vi "LoadArmValues.vi"(8 "error in (no error)":errorcluster, 11 "Robot":T1) -> (0 "error out":errorcluster)   [LabVIEW 2015]
uses:
  LowShooter/Implementation/Shooter Settings Type Def.ctl
  Drive/Implementation/Advanced Drive VIs/PID Type Def.ctl
  Arm/Arm Settings Type Def.ctl
  Robot Type Def.ctl
  <vilib>/Rock Robotics/Network Tables/NT Read Numeric Array.vi
  LowShooter/Implementation/Shooter Global.vi
panel:
  out "Arm Settings":T2
  out "PID":T3
  out "Shooter Settings":T4
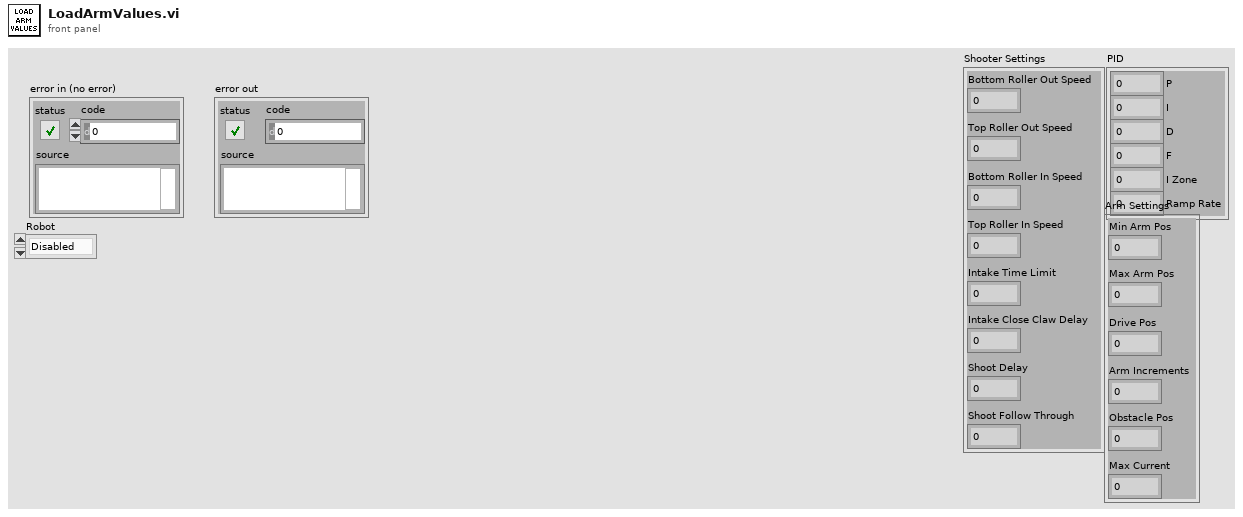
[diagram p1: front panel]
types:
  T1 = typedef "Robot Type Def.ctl" = enum32{"Disabled", "Ghost", "Casper", "Lofty", "Board", "RaceRobot", "Casper 2.0", "Excalibot 2.0"}
  T2 = typedef "Arm Settings Type Def.ctl" = cluster{"Min Arm Pos":dbl, "Max Arm Pos":dbl, "Drive Pos":dbl, "Arm Increments":dbl, "Obstacle Pos":dbl, "Max Current":dbl}
  T3 = typedef "PID Type Def.ctl" = cluster{"P":dbl, "I":dbl, "D":dbl, "F":dbl, "I Zone":dbl, "Ramp Rate":dbl}
  T4 = typedef "Shooter Settings Type Def.ctl" = cluster{"Bottom Roller Out Speed":dbl, "Top Roller Out Speed":dbl, "Bottom Roller In Speed":dbl, "Top Roller In Speed":dbl, "Intake Time Limit":dbl, "Intake Close Claw Delay":dbl, "Shoot Delay":dbl, "Shoot Follow Through":dbl}
  T5 = typedef "Detailed Motor Type Def.ctl" = cluster{"MotorRef":T6, "Encoder Ticks Per Rev":dbl, "Set Position":dbl, "Wheel Radius":dbl}
  T6 = typedef "WPI_MotorControlDeviceRef.ctl" = cluster{"DeviceStatus":errorcluster, "Type":T7, "PWM":cluster{"PWM Channel":T8, "DeadBand":T9}, "CAN":cluster{"Device Number":u8, "Control Mode":T10, "Semaphore":T11, "Max Vout":dbl, "TalonSRX Control Mode":T12}, "Invert":bool}
  T7 = typedef "WPI_MotorControlType.ctl" = enum16{"PWM", "CAN", "CANTalonSRX"}
  T8 = typedef "FPGA_DIOPWMChannel.ctl" = enum8{"PWM 0", "PWM 1", "PWM 2", "PWM 3", "PWM 4", "PWM 5", "PWM 6", "PWM 7", "PWM 8", "PWM 9", "PWM MXP 0", "PWM MXP 1", "PWM MXP 2", "PWM MXP 3", "PWM MXP 4", "PWM MXP 5", "PWM MXP 6", "PWM MXP 7", "PWM MXP 8", "PWM MXP 9", "Invalid"}
  T9 = typedef "WPI_PWMDeadband.ctl" = cluster{"Name":string, "maxPositivePwm":i32, "minPositivePwm":i32, "centerPwm":i32, "maxNegativePwm":i32, "minNegativePwm":i32, "angularRange":u16}
  T10 = typedef "WPI_CANJaguar_ControlMode.ctl" = enum8{"Percent VBus", "Current", "Speed", "Position", "Voltage"}
  T11 = typedef "Semaphore RefNum" = refnum<k1>
  T12 = typedef "WPI_CANTalonSRX_APIControlMode.ctl" = enum8{"Percent VBus", "Speed", "Position", "Slave", "Unchanged / Invalid", "Voltage Compensation", "Current", "Motion Profile"}
  T13 = typedef "WPI_CANTalonSRX_GlobalStatus.ctl" = cluster{"Applied Throttle":dbl, "Module Enabled":bool, "CAN Error":errorcluster, "Closed Loop Error":dbl, "Forward Limit Switch Closed":bool, "Reverse Limit Switch Closed":bool, "Sensor Position":dbl, "Sensor Velocity":dbl, "Current":dbl, "Sticky Fault - Over Temp":bool, "Sticky Fault - Under Voltage":bool, "Sticky Fault - Forward Limit":bool, "Sticky Fault - Reverse Limit":bool, "Sticky Fault - Forward Soft Limit":bool, "Sticky Fault - Reverse Soft Limit":bool, "Brake is Enabled":bool, "Encoder Position":dbl, "Encoder Velocity":dbl, "Encoder Index Count":dbl, "Encoder A Pin State":bool, "Encoder B Pin State":bool, "Encoder Index Pin State":bool, "Analog In":dbl, "Analog In Velocity":dbl, "Temperature (C)":dbl, "Battery Voltage":dbl, "Control 5 Is Supported":bool, "Current Profile Slot Select":dbl, "Pos Div 8":bool, "Vel Div 4":bool, "Pulse Width Position":i32, "Pulse Width Velocity":i32, "Pulse Width Rise To Rise (us)":i32, "Pulse Width Rise To Fall (us)":i32, "Mot Prof Active Is Under Run":bool, "Mot Prof Active Has Under Run":bool, "Mot Prof Active Is Last":bool, "Mot Prof Active Velocity Only":bool, "Mot Prof Active Is Valid":bool, "Mot Prof Buffer Is Full":bool, "Mot Prof Active Profile Slot Select":i32, "Mot Prof NextID":i32, "Mot Prof Count":i32, "Mot Prof Active Velocity":dbl, "Mot Prof Active Position":dbl, "Mot Prof Output Enable":i32}
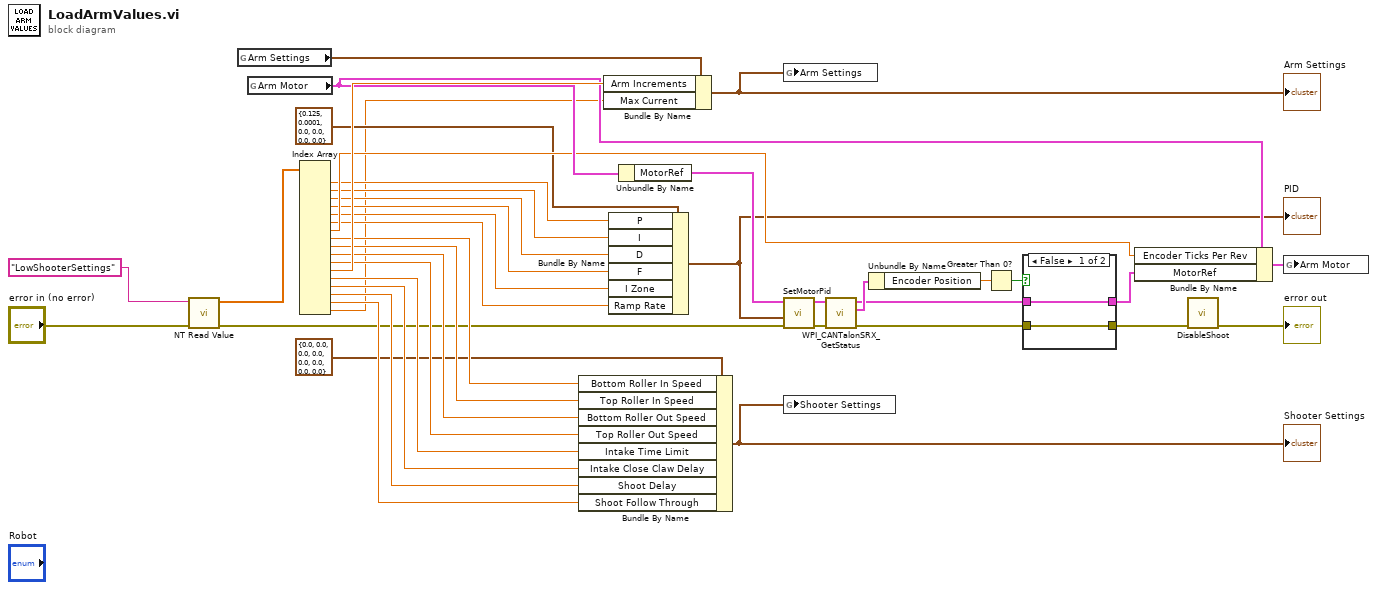
[diagram p0: block diagram]
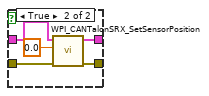
[diagram p2: hidden frame]
diagram:
  n1 = call-poly <vilib>:"NT Read Value.vi"("error in"="error in (no error)", "Name"="LowShooterSettings") -> ("error out"=w12:errorcluster, "Numeric Array"=w23:dbl[])  [unwired: 8 in]
  n2 = global read "Shooter Global.vi" "Arm Settings"() -> (w40:T2)
  n3 = global read "Shooter Global.vi" "Arm Motor"() -> (w36:T5)
  n4 = Index Array(array=w23) -> (element #1=w16:dbl, element #2=w17:dbl, element #3=w18:dbl, element #4=w19:dbl, element #5=w20:dbl, element #6=w21:dbl, element #7=w27:dbl, element #8=w28:dbl, element #9=w29:dbl, element #10=w30:dbl, element #11=w31:dbl, element #12=w38:dbl, element #13=w32:dbl, element #14=w33:dbl, element #15=w34:dbl, element #16=w35:dbl, element #17=w11:dbl)  [unwired: 17 in]
  n5 = Bundle By Name(cluster=T4 {"Bottom Roller Out Speed"=0.0, "Top Roller Out Speed"=0.0, "Bottom Roller In Speed"=0.0, "Top Roller In Speed"=0.0, "Intake Time Limit"=0.0, "Intake Close Claw Delay"=0.0, "Shoot Delay"=0.0, "Shoot Follow Through"=0.0} ("Shooter Settings"), "Bottom Roller In Speed"=w28, "Top Roller In Speed"=w29, "Bottom Roller Out Speed"=w30, "Top Roller Out Speed"=w31, "Intake Time Limit"=w32, "Intake Close Claw Delay"=w33, "Shoot Delay"=w34, "Shoot Follow Through"=w35) -> (w26:T4)
  "Shooter Settings" <- w26
  n6 = Bundle By Name(cluster=w40, "Arm Increments"=w38, "Max Current"=w11) -> (w39:T2)
  "Arm Settings" <- w39
  n7 = Bundle By Name(cluster=T3 {"P"=0.125, "I"=0.0001, "D"=0.0, "F"=0.0, "I Zone"=0.0, "Ramp Rate"=0.0} ("PID"), "P"=w16, "I"=w17, "D"=w18, "F"=w19, "I Zone"=w20, "Ramp Rate"=w21) -> (w22:T3)
  "PID" <- w22
  n8 = Unbundle By Name(w36) -> ("MotorRef"=w24:T6)
  n9 = global write "Shooter Global.vi" "Arm Settings"(w39) -> ()
  n10 = call "SetMotorPid.vi"("error in (no error)"=w12, "PID"=w22, "Motor Ref In"=w24) -> ("error out"=w4:errorcluster, "Motor Ref Out"=w10:T6)  [unwired: 7 in]
  n11 = global write "Shooter Global.vi" "Shooter Settings"(w26) -> ()
  n12 = call <vilib>:"WPI_CANTalonSRX_GetStatus.vi"("error in (no error)"=w4, "CAN Talon SRX Ref"=w10) -> ("error out"=w3:errorcluster, "Talon SRX Status"=w9:T13, "CAN Talon SRX Ref"=w6:T6)  [unwired: 7 in]
  n13 = Unbundle By Name(w9) -> ("Encoder Position"=w8:dbl)
  n14 = Greater Than 0?(x=w8) -> (x > 0?=w7:bool)
  n15 = case shown="False" w7 {
    tunnel: w6 -> [w42 w47]
    tunnel: [w42 w46] -> w5
    tunnel: [w41 w44] -> w2
    tunnel: w3 -> [w41 w43]
    frame False {
    }
    frame True {
      n16 = call <vilib>:"WPI_CANTalonSRX_SetSensorPosition.vi"("error in (no error)"=w43, "New Sensor Position"=0.0, "CAN Talon SRX Ref"=w47) -> ("error out"=w44:errorcluster, "CAN Talon SRX Ref"=w46:T6)  [unwired: 7 in]
    }
  }
  n17 = Bundle By Name(cluster=w36, "Encoder Ticks Per Rev"=w27, "MotorRef"=w5) -> (w37:T5)
  n18 = call "DisableShoot.vi"("error in (no error)"=w2) -> ("error out"=→"error out":errorcluster)  [unwired: 10 in]
  n19 = global write "Shooter Global.vi" "Arm Motor"(w37) -> ()
